vi "create 0mqPortNumbers.vi"(9 "level":u32 caption="level (0, 1, 2, or 3)" max=3, 10 "sysName":string) -> (0 "repPort":string, 1 "reqPort":string, 2 "subPort":string, 3 "pubPort":string)   [LabVIEW 2018]
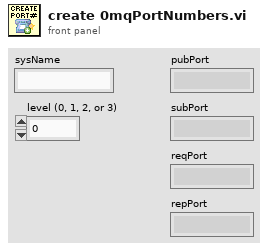
[diagram p1: front panel]
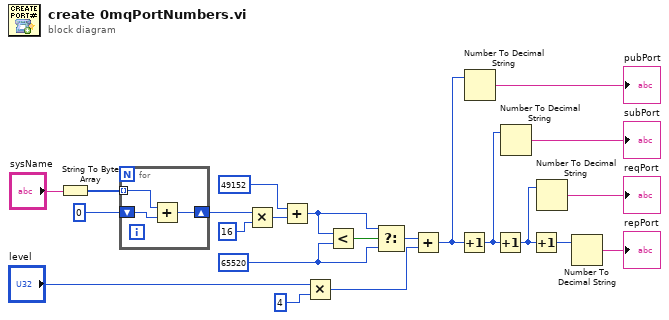
[diagram p0: block diagram]
diagram:
  w2 = u32 65520
  n1 = String To Byte Array(string="sysName") -> (unsigned byte array=w21:u8[])
  n2 = for {
    tunnel: w21 -> [w24] mode=indexing
    shift-right: [w25] -> w19
    shift-left: u32 0 -> [w23]
    n3 = Add(x=w24, y=w23) -> (x+y=w25:u32)
  }
  n4 = Multiply(x=w19, y=u32 16) -> (x*y=w9:u32)
  n5 = Add(x=u32 49152, y=w9) -> (x+y=w1:u32)
  n6 = Multiply(x="level", y=u32 4) -> (x*y=w6:u32)
  n7 = Less?(x=w1, y=w2) -> (x < y?=w3:bool)
  n8 = Select(t=w1, s=w3, f=w2) -> (s? t:f=w4:u32)
  n9 = Add(x=w4, y=w6) -> (x+y=w5:u32)
  n10 = Increment(x=w5) -> (x+1=w11:u32)
  n11 = Number To Decimal String(number=w5) -> (decimal integer string=→"pubPort":string)  [unwired: 1 in]
  n12 = Increment(x=w11) -> (x+1=w10:u32)
  n13 = Number To Decimal String(number=w11) -> (decimal integer string=→"subPort":string)  [unwired: 1 in]
  n14 = Increment(x=w10) -> (x+1=w12:u32)
  n15 = Number To Decimal String(number=w10) -> (decimal integer string=→"reqPort":string)  [unwired: 1 in]
  n16 = Number To Decimal String(number=w12) -> (decimal integer string=→"repPort":string)  [unwired: 1 in]
